vi "Ver 1.4.vi"() -> ()   [LabVIEW 2015]
uses:
  <instrlib>/Keithley 622x LV 2009/Configure/Source/Typedefs/KE622x -- Current Range.ctl
  <instrlib>/Keithley 622x LV 2009/Configure/Source/Typedefs/KE622x -- Current Ranges.ctl
  <instrlib>/Keithley 622x LV 2009/Typedefs/KE622x -- On Off Control.ctl
  <instrlib>/Keithley 622x LV 2009/Configure/Source/Typedefs/KE622x -- Voltage Limit.ctl
  <instrlib>/Keithley 622x LV 2009/Utility/Typedefs/KE622x -- Instrument Type.ctl
  <instrlib>/Keithley 2000/Public/Configure/Configure DC Volts.vi
  <userlib>/LV-Link3/PolySubVIs/DtCreateAinChan.vi
  <userlib>/LV-Link3/PolySubVIs/DtOLTimingSetInput.vi
  <userlib>/LV-Link3/PolySubVIs/DtOLReadMultiple2D.vi
  <instrlib>/Keithley 2000/Keithley 2000.lvlib
  <instrlib>/Keithley 622x LV 2009/Keithley 622x.lvlib
panel:
  in  "Stop Button":bool
  out "Acquired Data":dbl[][](graph)
  in  "Sample Rate":dbl=10000.0
  in  "Samples Per Channel":dbl=1000.0
  in  "Device":string(combo)
  in  "Channels":string="0"
  in  "Start Button":bool
  in  "Number \nof points":i32
  in  "Folder\nprename":string
  out "XY Graph":cluster{u32[], dbl[]}(graph)
  out "Measurement":dbl
  out "T0":u32
  out "LIMIT":bool
  out "LIMIT":bool
  out "Error Code":string
  in  "Comments":string
  out "file":refnum<file>
  out "2000":refnum<visa-resource-name>
  out "6221":refnum<visa-resource-name>
  out "Step  (A)":dbl=5e-05 format="%#_3p"
  in  "Stop\ncurrent (A)":dbl=0.002 format="%#_6p"
  in  "Start \ncurrent (A)":dbl=0.001 format="%#_6p"
  in  "Check For SCPI Errors? (T)":bool=TRUE
  out "Interlock Tripped?":bool
  out "Compliance?":bool
  in  "Turn Off Output \nIf Compliance?":bool=TRUE
  in  "Turning ON/OFF\ncurrent output":T1=enum."On"
  in  "Range Selection":T2={"Auto Range?"=TRUE, "Man / Selected\nRange"=enum."2nA"}
  # "FILE CONFIGURATION"
  # "ADMIN PANEL"
  # "KEITHLEY 6221 CONFIGURATION (ADMIN ONLY)"
  # "KEITHLEY DAQ CONFIGURATION (ADMIN ONLY)"
  # "I don't know what the hell it is,\njust don't touch it"
  # "START, STOP, STEP, CONFIGURATION"
  # "IF ON"
  # "Compliance = Limiting output voltage\nThis switch determines if we want to switch \noff the current output if wee exceed compliance"
  # "There is a safe switch at \nthe back of the instrument \nThis indicator shows if it is on"
  # "You have hit a damn jackpot \nby exceeding the limited voltage\nCongrats"
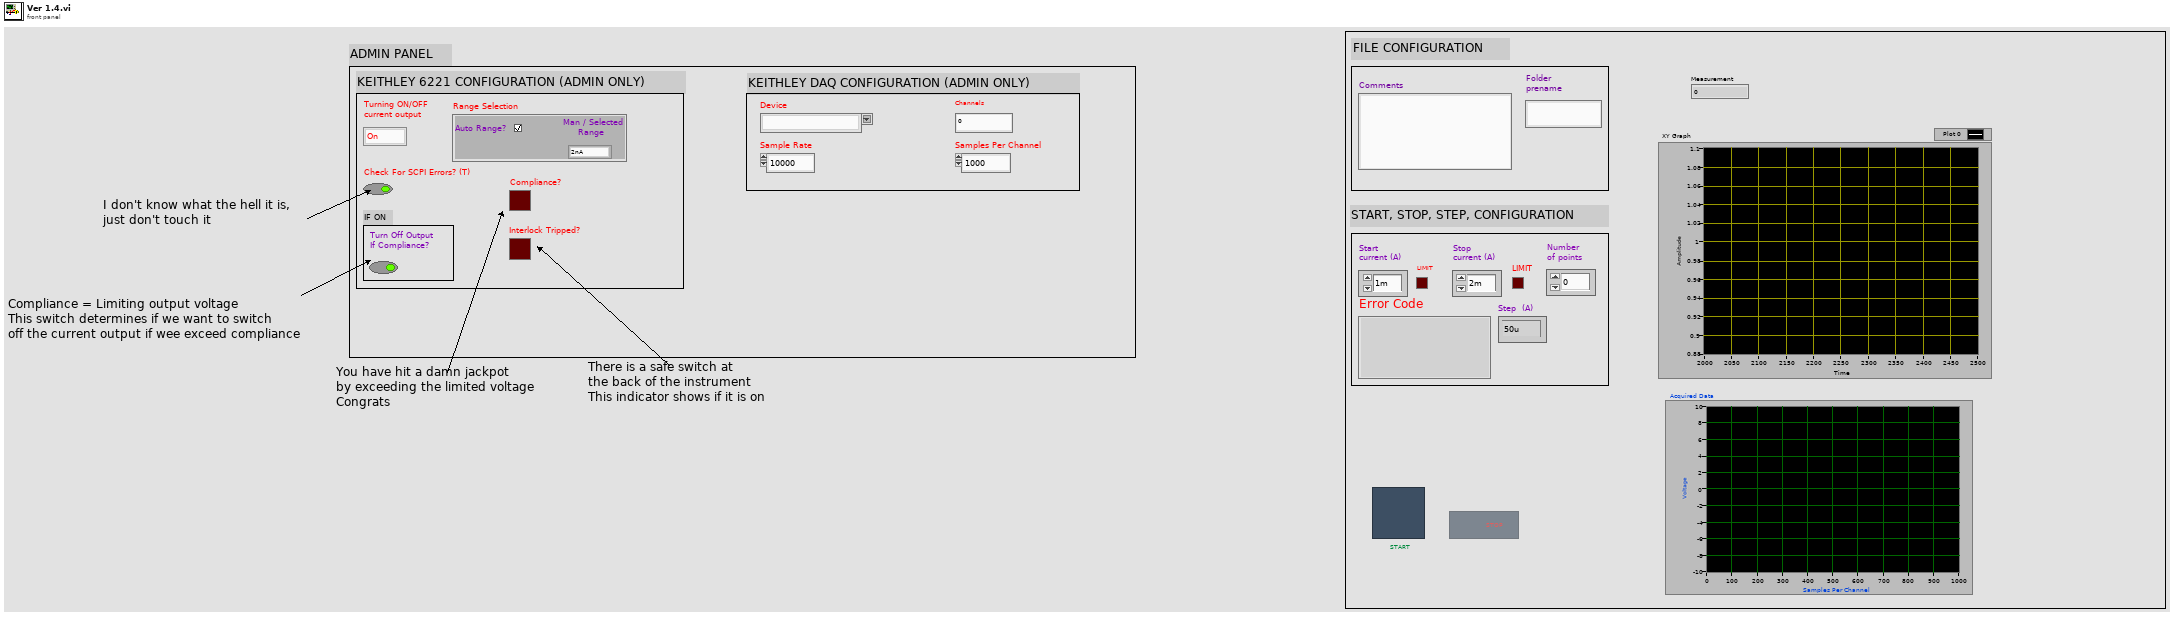
[diagram p1: front panel]
types:
  T1 = typedef "Keithley 622x.lvlib/KE622x -- On Off Control.ctl" = enum16{"Off", "On"}
  T2 = typedef "Keithley 622x.lvlib/KE622x -- Current Range.ctl" = cluster{"Auto Range?":bool, "Man / Selected\nRange":T3}
  T3 = typedef "Keithley 622x.lvlib/KE622x -- Current Ranges.ctl" = enum16{"2nA", "20nA", "200nA", "2uA", "20uA", "200uA", "2mA", "20mA", "100mA"}
  T4 = enum8{"Enabled", "Disabled", "Disabled and Grayed Out"}
  T5 = typedef "Keithley 622x.lvlib/KE622x -- Voltage Limit.ctl" = dbl
  T6 = typedef "Keithley 622x.lvlib/KE622x -- Instrument Type.ctl" = enum16{"KE6220", "KE6221"}
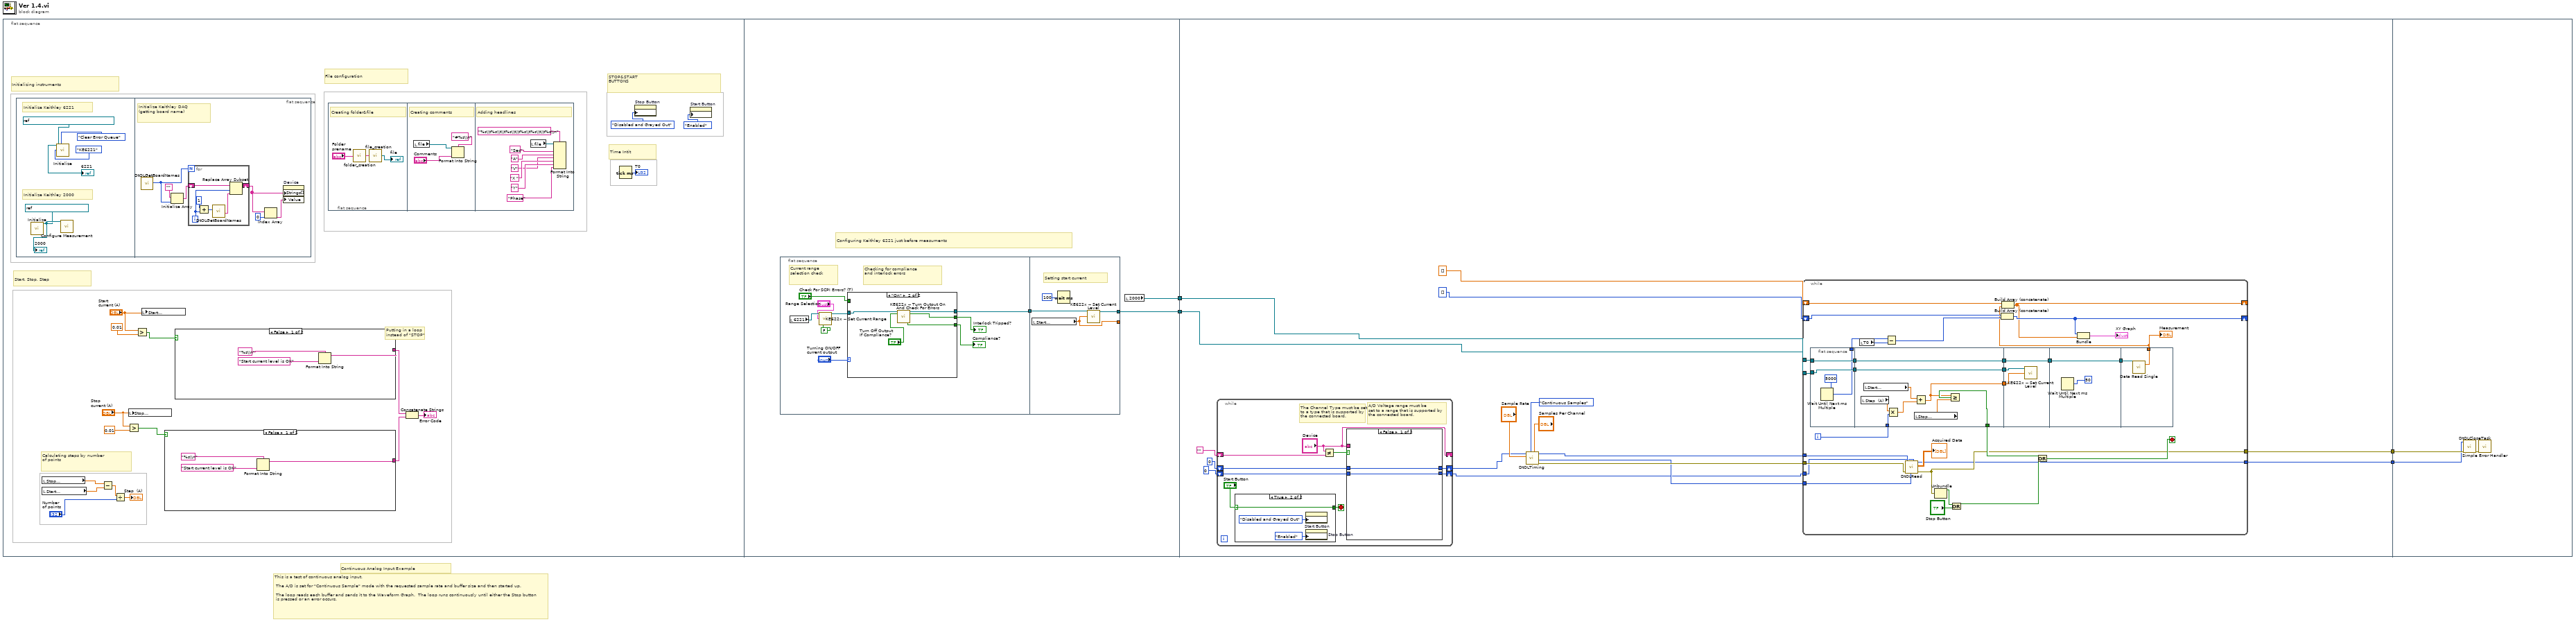
[diagram p0: block diagram]
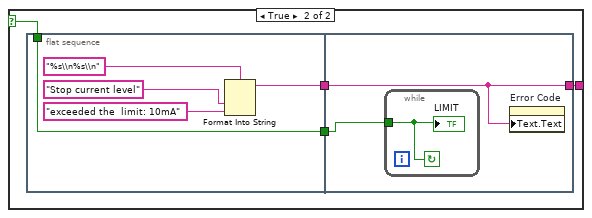
[diagram p2: hidden frame]
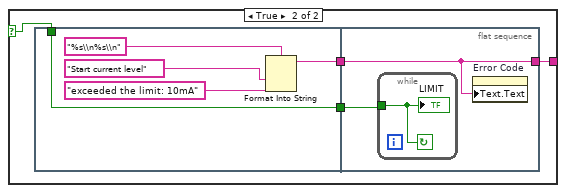
[diagram p3: hidden frame]
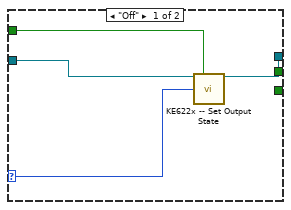
[diagram p4: hidden frame]
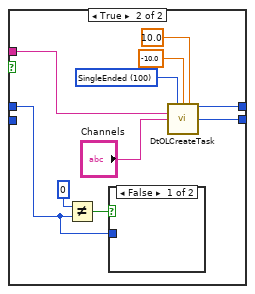
[diagram p6: hidden frame]
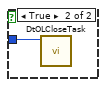
[diagram p7: hidden frame]
diagram:
  # "Continuous Analog Input Example"
  # "This is a test of continuous analog input. \n\n The A/D is set for \"Continuous Sample\" mode with the requested sample rate and buffer size and then started up.\n\n The loop reads each buffer and sends it to the Waveform Graph.  The loop runs continuously until either the Stop button\n is pressed or an error occurs."
  n1 = flat-sequence {
    tunnel: [w85] -> w4
    tunnel: [w84] -> w3
    tunnel: w4 -> [w119]
    tunnel: w3 -> [w118]
    tunnel: [w117] -> w2
    tunnel: [w116] -> w1
    tunnel: w2 -> [w204]
    tunnel: w1 -> [w203]
    frame #0 {
      # "STOP&START \nBUTTONS"
      # "Calculating steps by number\nof points"
      # "Time Intit"
      # "Putting in a loop \ninstead of \"STOP\""
      # "Start, Stop, Step"
      # "Initializing instruments"
      # "File configuration"
      n2 = flat-sequence {
        frame #0 {
          # "Initialize Keithley 2000"
          # "Initialize Keithley 6221"
          n3 = call <instrlib>:"Initialize.vi"("VISA resource name"=refnum<visa-resource-name> "KEITHLEY_MULTIMETER") -> ("VISA resource name out"=w23:refnum<visa-resource-name>)  [unwired: 17 in, 1 out]
          "2000" <- w23
          n4 = call <instrlib>:"Initialize.vi"("VISA resource name"=refnum<visa-resource-name> "KEITHLEY_DC_AC_CURRENT_SOURCE", "Error Queue Option"=enum16{"Clear Error Queue", "Error Query"}."Clear Error Queue", "Instrument Type"=KE622x_--_Instrument_Type."KE6221") -> ("VISA resource name out"=→"6221":refnum<visa-resource-name>)  [unwired: 11 in, 1 out]
          n5 = call-poly <instrlib>:"Configure Measurement.vi"("VISA resource name"=w23) -> ()  [unwired: 17 in, 2 out]
        }
        frame #1 {
          # "Initialize Keithley DAQ \n(getting board name)"
          n6 = call <userlib>:"DtOLGetBoardNames.vi"() -> ("Number of boards"=w28:u32)  [unwired: 9 in, 2 out]
          n7 = Initialize Array("", w28) -> (w30:string[])
          n8 = for {
            N: w28 -> [_]
            shift-right: [w36] -> w33
            shift-left: w30 -> [w37]
            i -> [w35]
            n9 = Add(x=1, y=w35) -> (x+y=w39:i32)
            n10 = call <userlib>:"DtOLGetBoardNames.vi"("Select Board"=w39) -> ("Board Name"=w34:string)  [unwired: 8 in, 2 out]
            n11 = Replace Array Subset(array=w37, new element=w34, index=w35) -> (w36:string[])
          }
          n12 = Index Array(array=w33, index=0) -> (element=w32:string)
          n13 = property on="Device" class="CmbBox"("Strings[]"=w33, "Value"=w32) -> ()  [unwired: 2 in, 2 out]
        }
      }
      n14 = local read "Stop\ncurrent (A)"() -> (w10:dbl)
      n15 = local read "Start \ncurrent (A)"() -> (w9:dbl)
      n16 = Subtract(x=w10, y=w9) -> (x-y=w7:dbl)
      n17 = Divide(x=w7, y="Number \nof points") -> (x/y=→"Step  (A)":dbl)
      n18 = Greater?(x="Stop\ncurrent (A)", y=T5 0.01) -> (0:w16:bool)
      n19 = local write "Stop\ncurrent (A)"("Stop\ncurrent (A)") -> ()
      n20 = Greater?(x="Start \ncurrent (A)", y=T5 0.01) -> (0:w17:bool)
      n21 = local write "Start \ncurrent (A)"("Start \ncurrent (A)") -> ()
      n22 = case shown="False" w16 {
        selector: w16 -> [_ w43]
        tunnel: [w40 w46] -> w14
        frame False {
          n23 = Format Into String(format string="%s\\n", "Start current level is OK" ("false string")) -> (resulting string=w40:string)  [unwired: 2 in, 1 out]
        }
        frame True {
          n24 = flat-sequence {
            tunnel: [w48] -> w45
            tunnel: [w47] -> w44
            tunnel: w43 -> [w47]
            tunnel: [w52] -> w46
            tunnel: w45 -> [w52]
            tunnel: w44 -> [w53]
            frame #0 {
              n25 = Format Into String(format string="%s\\n%s\\n", "Stop current level" ("String"), "exceeded the  limit: 10mA" ("input 2")) -> (resulting string=w48:string)  [unwired: 2 in, 1 out]
            }
            frame #1 {
              n26 = while {
                tunnel: w53 -> [w54]
                stop <- w54 continue-if-true
                "LIMIT" <- w54
              }
              n27 = property on="Error Code" class="Str"("Text.Text"=w52) -> ()  [unwired: 2 in, 2 out]
            }
          }
        }
      }
      n28 = case shown="False" w17 {
        selector: w17 -> [_ w59]
        tunnel: [w55 w61] -> w15
        frame False {
          n29 = Format Into String(format string="%s\\n", "Start current level is OK" ("false string")) -> (resulting string=w55:string)  [unwired: 2 in, 1 out]
        }
        frame True {
          n30 = flat-sequence {
            tunnel: [w63] -> w60
            tunnel: w59 -> [w62]
            tunnel: [w62] -> w58
            tunnel: [w67] -> w61
            tunnel: w60 -> [w67]
            tunnel: w58 -> [w68]
            frame #0 {
              n31 = Format Into String(format string="%s\\n%s\\n", "Start current level" ("String"), "exceeded the limit: 10mA" ("input 2")) -> (resulting string=w63:string)  [unwired: 2 in, 1 out]
            }
            frame #1 {
              n32 = while {
                tunnel: w68 -> [w69]
                stop <- w69 continue-if-true
                "LIMIT" <- w69
              }
              n33 = property on="Error Code" class="Str"("Text.Text"=w67) -> ()  [unwired: 2 in, 2 out]
            }
          }
        }
      }
      n34 = flat-sequence {
        frame #0 {
          # "Creating folder&file"
          n35 = call "folder_creation.vi"("Name"="Folder\nprename") -> ("String"=w71:string)
          n36 = call "file_creation.vi"("String"=w71) -> ("refnum out"=→"file":refnum<file>)
        }
        frame #1 {
          # "Creating comments"
          n37 = local read "file"() -> (w73:refnum<file>)
          n38 = Format Into String(format string="#%s\\n", initial string=w73, "Comments") -> ()  [unwired: 1 in, 2 out]
        }
        frame #2 {
          # "Adding headlines"
          n39 = local read "file"() -> (w83:refnum<file>)
          n40 = Format Into String(format string="%s\\t%s\\t\\t%s\\t\\t%s\\t%s\\t\\t%s\\n", initial string=w83, "Sec" ("input 1"), "A" ("input 2"), "V" ("input 3"), "X " ("input 3"), "Y" ("input 3"), "Phase" ("input 3")) -> ()  [unwired: 1 in, 2 out]
        }
      }
      n41 = Concatenate Strings(w15, w14) -> (→"Error Code":string)
      n42 = Tick Count (ms)() -> (millisecond timer value=→"T0":u32)
      n43 = property on="Stop Button" class="Bool"("DisabledEnum"=T4."Disabled and Grayed Out" ("Disabled")) -> ()  [unwired: 2 in, 2 out]
      n44 = property on="Start Button" class="Bool"("DisabledEnum"=T4."Enabled" ("Disabled")) -> ()  [unwired: 2 in, 2 out]
    }
    frame #1 {
      # "Configuring Keithley 6221 just before measuments"
      n45 = flat-sequence {
        tunnel: [w87] -> w86
        tunnel: [w105] -> _
        tunnel: [w107] -> w84
        tunnel: w86 -> [w106]
        frame #0 {
          # "Current range \nselection check"
          # "Checking for compliance\nand interlock errors"
          n46 = local read "6221"() -> (w90:refnum<visa-resource-name>)
          n47 = call <instrlib>:"KE622x -- Set Current Range.vi"("Resource In"=w90, "Current Range In"="Range Selection", "Read Back Set Values? (T)"=FALSE) -> ("Resource Out (dupl)"=w95:refnum<visa-resource-name>)  [unwired: 10 in, 2 out]
          n48 = case shown="\"On\"" "Turning ON/OFF\ncurrent output" {
            selector: "Turning ON/OFF\ncurrent output" -> [w99 _]
            tunnel: [_ w103] -> w93
            tunnel: [_ w102] -> w94
            tunnel: "Check For SCPI Errors? (T)" -> [w98 _]
            tunnel: w95 -> [w96 w101]
            tunnel: [w97 w100] -> w87
            frame "Off" {
              n49 = call <instrlib>:"KE622x -- Set Output State.vi"("Resource In"=w96, "Check For SCPI Errors? (T)"=w98, "Output State"=w99) -> ("Resource Out (dupl)"=w97:refnum<visa-resource-name>)  [unwired: 11 in, 1 out]
            }
            frame "On" {
              n50 = call <instrlib>:"KE622x -- Turn Output On And Check For Errors.vi"("Resource In"=w101, "Turn Off Output If Compliance?"="Turn Off Output \nIf Compliance?") -> ("Resource Out (dupl)"=w100:refnum<visa-resource-name>, "Interlock Tripped?"=w103:bool, "Compliance?"=w102:bool)  [unwired: 10 in, 1 out]
            }
          }
          "Interlock Tripped?" <- w93
          "Compliance?" <- w94
        }
        frame #1 {
          # "Setting start current"
          n51 = local read "Start \ncurrent (A)"() -> (w105:dbl)
          n52 = Wait (ms)(milliseconds to wait=u32 100) -> ()  [unwired: 1 out]
          n53 = call <instrlib>:"KE622x -- Set Current Level.vi"("Resource In"=w106, "Current Level (A) In"=w105) -> ("Resource Out (dupl)"=w107:refnum<visa-resource-name>)  [unwired: 12 in, 1 out]
        }
      }
      n54 = local read "2000"() -> (w85:refnum<visa-resource-name>)
    }
    frame #2 {
      n55 = while {
        shift-right: ["Device"] -> _
        shift-left: "" -> [w184]
        shift-right: [w181] -> w122
        shift-left: 0 ("Task out") -> [w182]
        shift-right: [w179] -> w112
        shift-left: 0 ("Task out") -> [w178]
        stop <- w180 stop-if-true
        # "The Channel Type must be set\nto a type that is supported by \nthe connected board."
        # "A/D Voltage range must be\nset to a range that is supported by \nthe connected board."
        n56 = case shown="True" "Start Button" {
          selector: "Start Button" -> [w186 w189]
          tunnel: [w186 w189] -> w180
          frame False {
          }
          frame True {
            n57 = property on="Start Button" class="Bool"("DisabledEnum"=T4."Disabled and Grayed Out" ("Disabled")) -> ()  [unwired: 2 in, 2 out]
            n58 = property on="Stop Button" class="Bool"("DisabledEnum"=T4."Enabled" ("Disabled")) -> ()  [unwired: 2 in, 2 out]
          }
        }
        n59 = Not Equal?(x="Device", y=w184) -> (x != y?=w185:bool)
        n60 = case shown="False" w185 {
          tunnel: "Device" -> [_ w198]
          tunnel: [w191 w197] -> w181
          tunnel: w182 -> [w191 w194]
          tunnel: [w190 w192] -> w179
          tunnel: w178 -> [w190 _]
          frame False {
          }
          frame True {
            w199 = 100 items=["SingleEnded"=100, "Differential"=101] ("Channel Type")
            n61 = Not Equal?(x=0, y=w194) -> (x != y?=w195:bool)
            n62 = case shown="False" w195 {
              tunnel: w194 -> [_ w202]
              frame False {
              }
              frame True {
                n63 = call <userlib>:"DtOLCloseTask.vi"("Task in"=w202) -> ()  [unwired: 10 in, 1 out]
              }
            }
            n64 = call-poly <userlib>:"DtOLCreateTask.vi"("Channel Type"=w199, "Range Min"=-10.0, "Range Max"=10.0, "Board Name"=w198, "Channel"="Channels") -> ("Task out"=w197:i32, "Actual Number of Channels"=w192:u32)  [unwired: 8 in, 1 out]
          }
        }
      }
      n65 = call-poly <userlib>:"DtOLTiming.vi"("Samples Per Channel"="Samples Per Channel", "Sample Mode"=enum16{"Finite Samples", "Continuous Samples"}."Continuous Samples", "Sample Freq (Hz)"="Sample Rate", "Task in"=w122) -> ("error out"=w115:errorcluster, "Buffer Size"=w114:u32, "Task out"=w113:i32)  [unwired: 4 in, 1 out]
      n66 = while {
        shift-right: [w138] -> _
        shift-left: dbl[] [] -> [w155]
        shift-right: [w139] -> _
        shift-left: i32[] [] -> [w154]
        tunnel: w119 -> [w151]
        tunnel: w118 -> [w149]
        tunnel: [w131] -> w117
        tunnel: [w130] -> w116
        tunnel: w115 -> [w129]
        tunnel: w114 -> [w128]
        tunnel: w113 -> [w127]
        tunnel: w112 -> [w126]
        i -> [w145]
        stop <- w132 stop-if-true
        n67 = flat-sequence {
          tunnel: w151 -> [w160]
          tunnel: [w160] -> w150
          tunnel: w149 -> [w159]
          tunnel: [w159] -> w148
          tunnel: [w157] -> w147
          tunnel: [w169] -> w144
          tunnel: w150 -> [w169]
          tunnel: w148 -> [w164]
          tunnel: w145 -> [w166]
          tunnel: [w162] -> w133
          tunnel: [w161] -> w142
          tunnel: [w164] -> w141
          tunnel: w144 -> [w172]
          tunnel: [w172] -> w143
          tunnel: w142 -> [w171]
          tunnel: w141 -> [w170]
          tunnel: w143 -> [w174]
          tunnel: [w174] -> w146
          tunnel: w146 -> [w176]
          tunnel: [w175] -> w140
          frame #0 {
            n68 = Wait Until Next ms Multiple(millisecond multiple=u32 5000) -> (millisecond timer value=w157:u32)
          }
          frame #1 {
            n69 = local read "Step  (A)"() -> (w167:dbl)
            n70 = local read "Start \ncurrent (A)"() -> (w168:dbl)
            n71 = Multiply(x=w167, y=w166) -> (x*y=w165:dbl)
            n72 = local read "Stop\ncurrent (A)"() -> (w163:dbl)
            n73 = Add(x=w168, y=w165) -> (x+y=w161:dbl)
            n74 = Greater Or Equal?(x=w161, y=w163) -> (x >= y?=w162:bool)
          }
          frame #2 {
            n75 = call <instrlib>:"KE622x -- Set Current Level.vi"("Resource In"=w170, "Current Level (A) In"=w171) -> ()  [unwired: 12 in, 2 out]
          }
          frame #3 {
            n76 = Wait Until Next ms Multiple(millisecond multiple=u32 50) -> ()  [unwired: 1 out]
          }
          frame #4 {
            n77 = call <instrlib>:"Data Read Single.vi"("VISA resource name"=w176) -> ("Measurement"=w175:dbl)  [unwired: 14 in, 4 out]
          }
        }
        n78 = local read "T0"() -> (w153:u32)
        n79 = Subtract(x=w147, y=w153) -> (x-y=w152:u32)
        n80 = call-poly <userlib>:"DtOLRead.vi"("Number Chan to Read"=w126, "Buffer size"=w128, "error in (no error)"=w129, "Task in"=w127) -> ("error out"=w131:errorcluster, "2D Data out"=→"Acquired Data":dbl[][], "Task out"=w130:i32)  [unwired: 3 in, 2 out]
        n81 = Unbundle(w131) -> ("status"=w137:bool)  [unwired: 2 out]
        n82 = Or(x=w137, y="Stop Button") -> (x .or. y?=w134:bool)
        n83 = Build Array (concatenate)(w154, w152) -> (w139:u32[])
        n84 = Build Array (concatenate)(w155, w140) -> (w138:dbl[])
        n85 = Or(x=w133, y=w134) -> (x .or. y?=w132:bool)
        n86 = Bundle(w139, w138) -> (→"XY Graph":cluster{u32[], dbl[]})  [unwired: 1 in]
        "Measurement" <- w140
      }
    }
    frame #3 {
      n87 = call <userlib>:"DtOLCloseTask.vi"("Error in"=w204, "Task in"=w203) -> ("Error Out"=w205:errorcluster)  [unwired: 9 in]
      n88 = call <vilib>:"Simple Error Handler.vi"("error in (no error)"=w205) -> ()  [unwired: 4 in, 5 out]
    }
  }
